vi "Attenuator Configuration.vi"(6 "Write? (f)":bool, 7 "Connection Refnum":T2, 8 "error in (no error)":errorcluster, 9 "Configuration (\"\")":string, 11 "Template Keys (empty)":T1) -> (0 "error out":errorcluster, 1 "Configuration":string, 3 "Template Keys":T1, 5 "Connection Refnum":T2)   [LabVIEW 2011]
uses:
  SI.LIB/ODBC/SQL Controls/Connection Refnum.ctl
  Addons/internet/utils/keyedarr.llb/Keyed Array.ctl
  Addons/internet/utils/strutil.llb/Case Matching.ctl
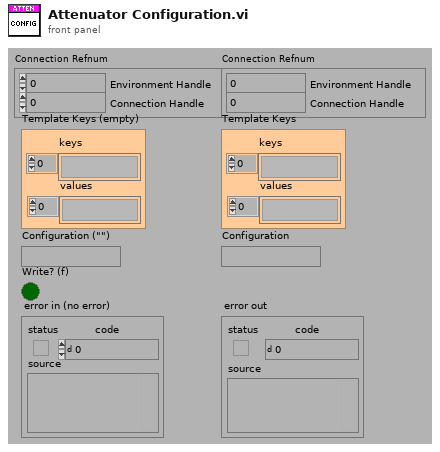
[diagram p1: front panel]
types:
  T1 = typedef "Keyed Array.ctl" = cluster{"keys":string[], "values":string[]}
  T2 = typedef "Connection Refnum.ctl" = cluster{"Environment Handle":i32, "Connection Handle":i32}
  T3 = typedef "Case Matching.ctl" = enum16{"a != A", "a == A", "system"}
  T4 = typedef "Attenuator Test Parameters.ctl" = cluster{"Stimulus":T5, "Measurement":T10, "Limit":T11, "Normalization":T12}
  T5 = typedef "Attenuator Stimulus Parameters.ctl" = cluster{"ATT Stimulus":T6, "VNA Stimulus":T7}
  T6 = typedef "Attenuator ATT Stimulus.ctl" = cluster{"Normalize":bool, "Value (dB)":dbl}
  T7 = typedef "Attenuator VNA Stimulus.ctl" = cluster{"Use Instrument Settings":bool, "Blank Frequencies":bool, "Sweep Type":enum32{"Linear", "Logarithmic", "List", "Power", "CW"}, "Sweep":cluster{"Fstart":dbl, "Fstop":dbl, "Units":T8, "Points":i32}, "Power (dBm)":dbl, "IFBW (Hz)":dbl, "Sweep Time (s)":dbl, "Calibration":T9}
  T8 = typedef "SP Frequency Units.ctl" = enum16{"Hz", "kHz", "MHz", "GHz", "Points"}
  T9 = typedef "Attenuator VNA Calibration State.ctl" = cluster{"State":bool, "String":string}
  T10 = typedef "Attenuator Measurement Cluster.ctl" = cluster{"Step (dB)":enum16{"0.25", "0.50", "1.00"}, "Start (dB)":dbl, "Stop (dB)":dbl}
  T11 = typedef "Attenuator Limit.ctl" = cluster{"Maximum Error":dbl}
  T12 = typedef "Attenuator Calibration State.ctl" = cluster{"Normalized?":bool, "Normalization Values (dB)":dbl[]}
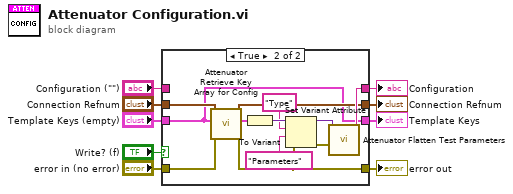
[diagram p0: block diagram]
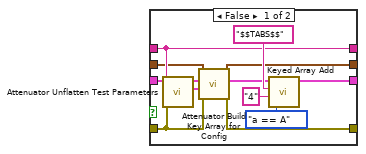
[diagram p2: hidden frame]
diagram:
  n1 = case shown="True" "Write? (f)" {
    tunnel: "error in (no error)" -> [w10 w27]
    tunnel: [w14 w22] -> w8
    tunnel: "Template Keys (empty)" -> [w12 w22]
    tunnel: "Configuration (\"\")" -> [w18 _]
    tunnel: [w13 w26] -> w5
    tunnel: [w18 w28] -> w4
    tunnel: "Connection Refnum" -> [w17 w25]
    tunnel: [w16 w24] -> w1
    frame False {
      n2 = call "Attenuator Unflatten Test Parameters.vi"("error in (no error)"=w10, "Parameter String"=w18) -> ("Attenuator Test Parameters"=w11:T4)  [unwired: 9 out]
      n3 = call "Attenuator Build Key Array for Config.vi"("error in (no error)"=w10, "DC Attenuation Test Parameters"=w11, "Key Array In"=w12, "Connection Refnum"=w17) -> ("error out"=w13:errorcluster, "Key Array Out"=w15:T1, "Connection Refnum"=w16:T2)  [unwired: 5 out]
      n4 = call "Keyed Array Add.vi"("case matching (sensitive)"=Case_Matching."a == A", "value"="4", "key"="$$TABS$$", "array in"=w15) -> ("array out"=w14:T1)  [unwired: 3 out]
    }
    frame True {
      n5 = call "Attenuator Retrieve Key Array for Config.vi"("error in (no error)"=w27, "Key Array In"=w22, "Connection Refnum"=w25) -> ("error out"=w26:errorcluster, "Attenuator Test Parameters"=w23:T4, "Connection Refnum"=w24:T2)  [unwired: 1 in, 5 out]
      n6 = To Variant(anything=w23) -> (Variant=w33:variant)
      n7 = Set Variant Attribute(Variant=w33, name="Type", value="Parameters" ("name"), error in=w26) -> (Variant out=w29:variant, error out=w32:errorcluster)  [unwired: 1 out]
      n8 = call "Attenuator Flatten Test Parameters.vi"("error in (no error)"=w32, "Parameter Variant"=w29) -> ("Parameter String"=w28:string)  [unwired: 9 out]
    }
  }
  "error out" <- w5
  "Connection Refnum" <- w1
  "Template Keys" <- w8
  "Configuration" <- w4
